vi "Convert Write ERD List to Message.vi"(0 "GEA Inputs":T1 {"Destination" format="%.0x"; "Source" format="%.0x"}, 7 "Write ERD List":T3(array[cluster]) {"ERD Number" format="%.0x"}, 11 "Error In":errorcluster) -> (4 "GEA Message":T2 {"Command" format="%02x"; "Destination" format="%02x"; "Source" format="%02x"}, 15 "Error Out":errorcluster)   [LabVIEW 2023]
doc: "This vi uses the Source / Destination from the GEA input and the ERD Write list to format a single GEA2 message to read the list of ERDs."
uses:
  type defs/Data In.ctl
  type defs/Source_Destination.ctl
  <vilib>/regexp/Match Regular Expression.xnode
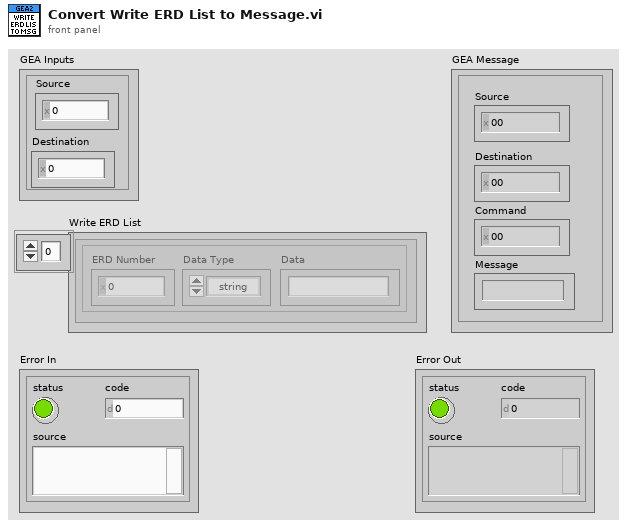
[diagram p1: front panel]
types:
  T1 = typedef "Source_Destination.ctl" = cluster{"Source":u8, "Destination":u8}
  T2 = typedef "Data In.ctl" = cluster{"Source":u8, "Destination":u8, "Command":u8, "Message":string}
  T3 = cluster{"ERD Number":u16, "Data Type":enum16{"string", "boolean", "uint8_t", "uint16_t", "uint32_t", "uint64_t", "int8_t", "int16_t", "int32_t", "int64_t"}, "Data":string}[]
  T4 = enum16{"string", "boolean", "uint8_t", "uint16_t", "uint32_t", "uint64_t", "int8_t", "int16_t", "int32_t", "int64_t"}
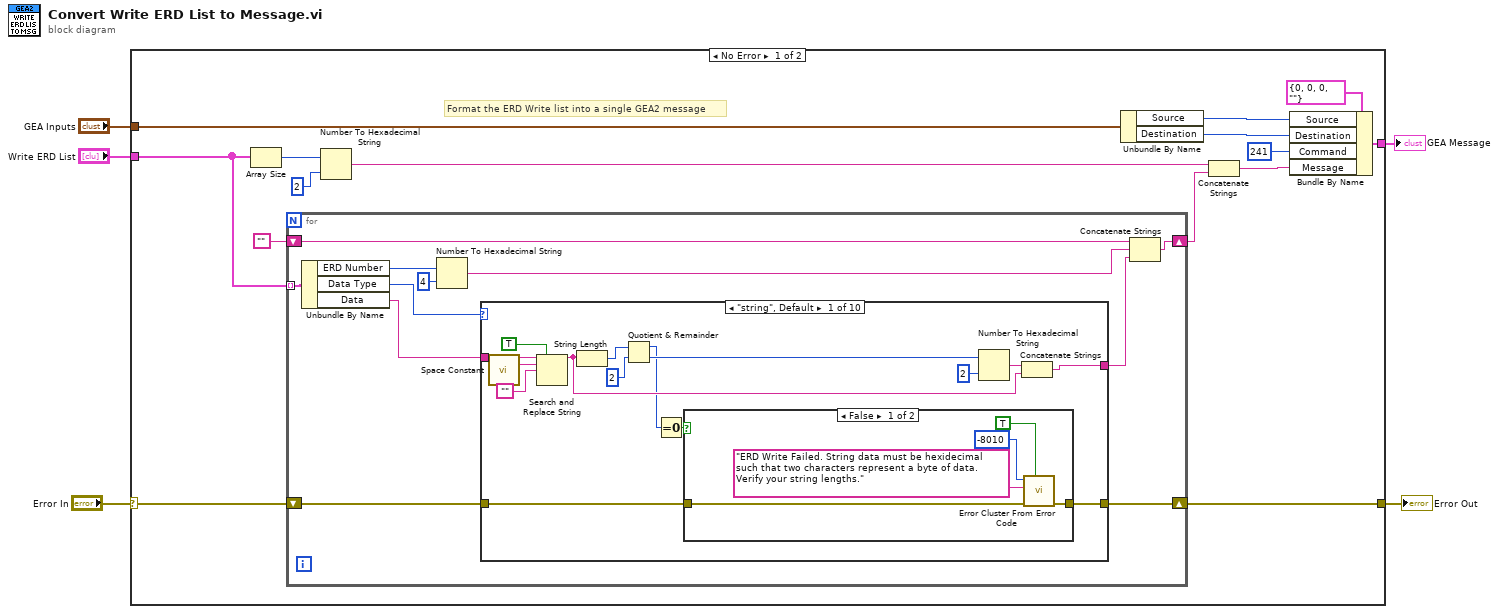
[diagram p0: block diagram]
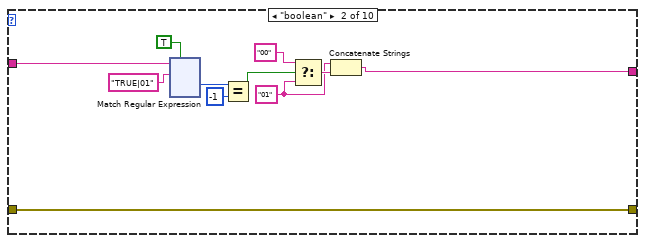
[diagram p3: hidden frame]
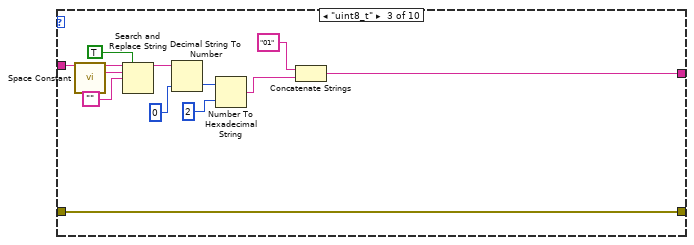
[diagram p4: hidden frame]
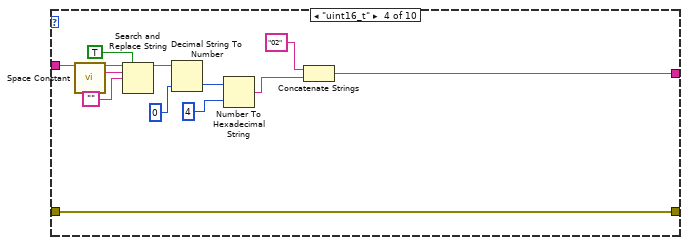
[diagram p5: hidden frame]
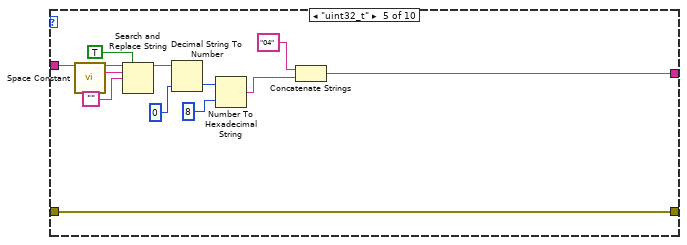
[diagram p6: hidden frame]
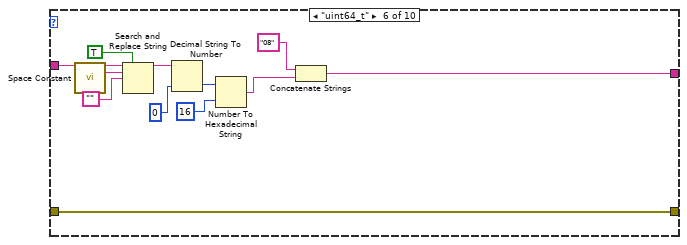
[diagram p7: hidden frame]
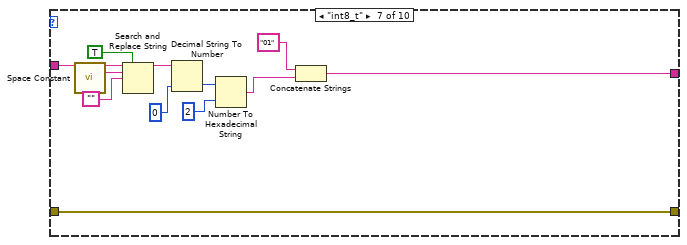
[diagram p8: hidden frame]
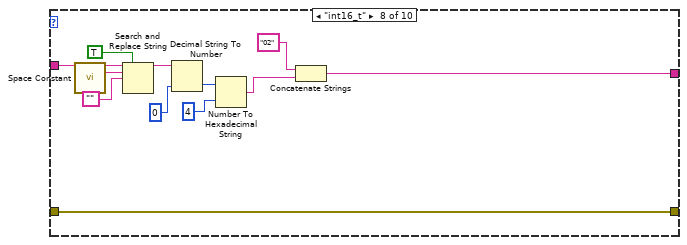
[diagram p9: hidden frame]
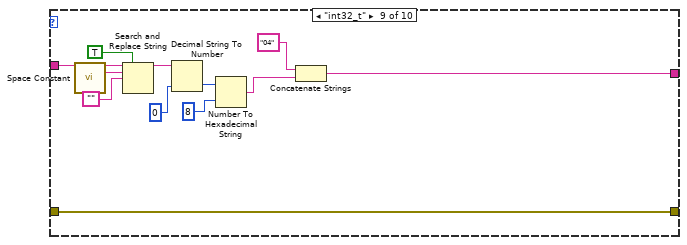
[diagram p10: hidden frame]
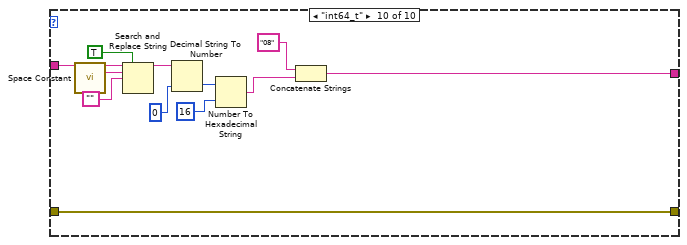
[diagram p11: hidden frame]
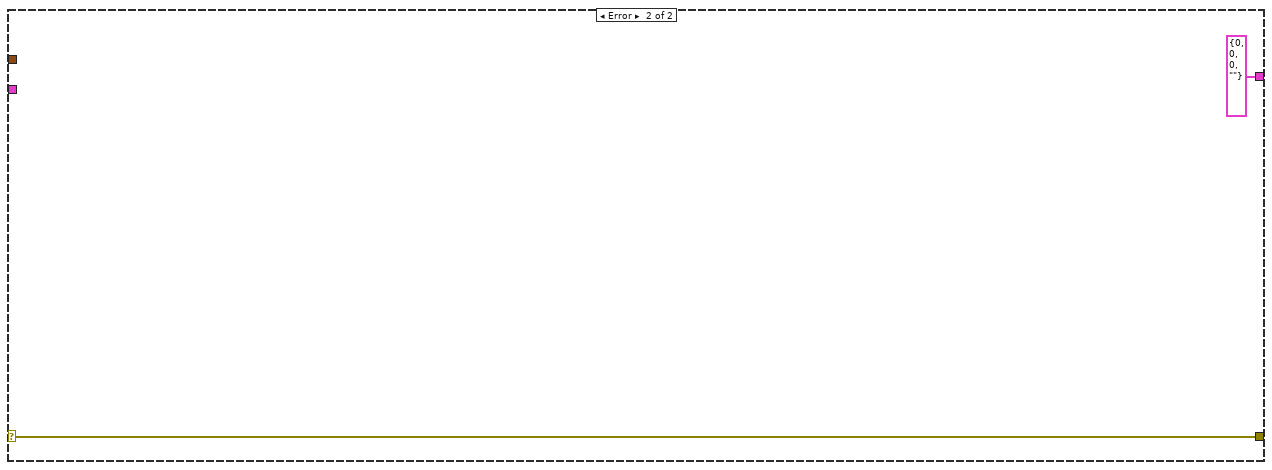
[diagram p12: hidden frame]
diagram:
  n1 = case shown="No Error" "Error In" {
    selector: "Error In" -> [w7 w278]
    tunnel: "Write ERD List" -> [w17 _]
    tunnel: "GEA Inputs" -> [w13 _]
    tunnel: [w8 T2 {"Source"=0, "Destination"=0, "Command"=0, "Message"=""} ("GEA Message")] -> w3
    tunnel: [w6 w278] -> w1
    frame No Error {
      # "Format the ERD Write list into a single GEA2 message"
      n2 = Array Size(array=w17) -> (size(s)=w19:i32)
      n3 = for {
        tunnel: w17 -> [w31] mode=indexing
        shift-right: [w26] -> w15
        shift-left: "" -> [w28]
        shift-right: [w21] -> w6
        shift-left: w7 -> [w22]
        n4 = Unbundle By Name(w31) -> ("ERD Number"=w30:u16, "Data Type"=w25:T4, "Data"=w24:string)
        n5 = Number To Hexadecimal String(1:i16 4 ("width (-)"), 2:w30) -> (0:w27:string)
        n6 = case shown="\"string\", Default" w25 {
          tunnel: w24 -> [w46 w62 w189 w194 w207 w219 w231 w243 w255 w267]
          tunnel: [w41 w55 w188 w195 w206 w218 w230 w242 w254 w266] -> w23
          tunnel: w22 -> [w35 w53 w181 w193 w205 w217 w229 w241 w253 w265]
          tunnel: [w32 w53 w181 w193 w205 w217 w229 w241 w253 w265] -> w21
          frame "string", Default {
            n7 = call <vilib>:"Space Constant.vi"() -> ("String"=w44:string)
            n8 = Search and Replace String(replace all?=TRUE ("replace all? (F)"), input string=w46, search string=w44, replace string="") -> (result string=w40:string)  [unwired: 4 in, 3 out]
            n9 = String Length(string=w40) -> (length=w38:i32)
            n10 = Quotient & Remainder(x=w38, y=2) -> (x-y*floor(x/y)=w34:i32, floor(x/y)=w37:i32)
            n11 = Equal To 0?(x=w34) -> (x = 0?=w33:bool)
            n12 = case shown="False" w33 {
              tunnel: w35 -> [w51 w52]
              tunnel: [w47 w52] -> w32
              frame False {
                n13 = call <vilib>:"Error Cluster From Error Code.vi"("show call chain? (False)"=TRUE, "error in (no error)"=w51, "error message (\"\")"="ERD Write Failed. String data must be hexidecimal such that two characters represent a byte of data. Verify your string lengths." ("error message (\"\")"), "error code (0)"=-8010) -> ("error out"=w47:errorcluster)  [unwired: 5 in]
              }
              frame True {
              }
            }
            n14 = Number To Hexadecimal String(1:i16 2 ("width (-)"), 2:w37) -> (0:w42:string)
            n15 = Concatenate Strings(w42, w40) -> (w41:string)
          }
          frame "boolean" {
            w54 = "01"
            n16 = xnode "Match Regular Expression"("input string"=w62, "regular expression"="TRUE|01", "ignore case? (F)"=TRUE) -> ("offset past match"=w60:i32)  [unwired: 3 in, 4 out]
            n17 = Equal?(x=w60, y=-1) -> (x = y?=w57:bool)
            n18 = Select(t="00", s=w57, f=w54) -> (s? t:f=w56:string)
            n19 = Concatenate Strings(w54, w56) -> (w55:string)
          }
          frame "uint8_t" {
            n20 = call <vilib>:"Space Constant.vi"() -> ("String"=w191:string)
            n21 = Search and Replace String(replace all?=TRUE ("replace all? (F)"), input string=w189, search string=w191, replace string="") -> (result string=w186:string)  [unwired: 4 in, 3 out]
            n22 = Decimal String To Number(string=w186, default (0L)=u8 0) -> (number=w183:u8)  [unwired: 1 in, 1 out]
            n23 = Number To Hexadecimal String(1:i16 2 ("width (-)"), 2:w183) -> (0:w182:string)
            n24 = Concatenate Strings("01", w182) -> (w188:string)
          }
          frame "uint16_t" {
            n25 = call <vilib>:"Space Constant.vi"() -> ("String"=w203:string)
            n26 = Search and Replace String(replace all?=TRUE ("replace all? (F)"), input string=w194, search string=w203, replace string="") -> (result string=w200:string)  [unwired: 4 in, 3 out]
            n27 = Decimal String To Number(string=w200, default (0L)=u16 0) -> (number=w197:u16)  [unwired: 1 in, 1 out]
            n28 = Number To Hexadecimal String(1:i16 4 ("width (-)"), 2:w197) -> (0:w196:string)
            n29 = Concatenate Strings("02", w196) -> (w195:string)
          }
          frame "uint32_t" {
            n30 = call <vilib>:"Space Constant.vi"() -> ("String"=w215:string)
            n31 = Search and Replace String(replace all?=TRUE ("replace all? (F)"), input string=w207, search string=w215, replace string="") -> (result string=w212:string)  [unwired: 4 in, 3 out]
            n32 = Decimal String To Number(string=w212, default (0L)=u32 0) -> (number=w209:u32)  [unwired: 1 in, 1 out]
            n33 = Number To Hexadecimal String(1:i16 8 ("width (-)"), 2:w209) -> (0:w208:string)
            n34 = Concatenate Strings("04", w208) -> (w206:string)
          }
          frame "uint64_t" {
            n35 = call <vilib>:"Space Constant.vi"() -> ("String"=w227:string)
            n36 = Search and Replace String(replace all?=TRUE ("replace all? (F)"), input string=w219, search string=w227, replace string="") -> (result string=w224:string)  [unwired: 4 in, 3 out]
            n37 = Decimal String To Number(string=w224, default (0L)=u64 0) -> (number=w221:u64)  [unwired: 1 in, 1 out]
            n38 = Number To Hexadecimal String(1:i16 16 ("width (-)"), 2:w221) -> (0:w220:string)
            n39 = Concatenate Strings("08", w220) -> (w218:string)
          }
          frame "int8_t" {
            n40 = call <vilib>:"Space Constant.vi"() -> ("String"=w239:string)
            n41 = Search and Replace String(replace all?=TRUE ("replace all? (F)"), input string=w231, search string=w239, replace string="") -> (result string=w236:string)  [unwired: 4 in, 3 out]
            n42 = Decimal String To Number(string=w236, default (0L)=i8 0) -> (number=w233:i8)  [unwired: 1 in, 1 out]
            n43 = Number To Hexadecimal String(1:i16 2 ("width (-)"), 2:w233) -> (0:w232:string)
            n44 = Concatenate Strings("01", w232) -> (w230:string)
          }
          frame "int16_t" {
            n45 = call <vilib>:"Space Constant.vi"() -> ("String"=w251:string)
            n46 = Search and Replace String(replace all?=TRUE ("replace all? (F)"), input string=w243, search string=w251, replace string="") -> (result string=w248:string)  [unwired: 4 in, 3 out]
            n47 = Decimal String To Number(string=w248, default (0L)=i16 0) -> (number=w245:i16)  [unwired: 1 in, 1 out]
            n48 = Number To Hexadecimal String(1:i16 4 ("width (-)"), 2:w245) -> (0:w244:string)
            n49 = Concatenate Strings("02", w244) -> (w242:string)
          }
          frame "int32_t" {
            n50 = call <vilib>:"Space Constant.vi"() -> ("String"=w263:string)
            n51 = Search and Replace String(replace all?=TRUE ("replace all? (F)"), input string=w255, search string=w263, replace string="") -> (result string=w260:string)  [unwired: 4 in, 3 out]
            n52 = Decimal String To Number(string=w260, default (0L)=0) -> (number=w257:i32)  [unwired: 1 in, 1 out]
            n53 = Number To Hexadecimal String(1:i16 8 ("width (-)"), 2:w257) -> (0:w256:string)
            n54 = Concatenate Strings("04", w256) -> (w254:string)
          }
          frame "int64_t" {
            n55 = call <vilib>:"Space Constant.vi"() -> ("String"=w275:string)
            n56 = Search and Replace String(replace all?=TRUE ("replace all? (F)"), input string=w267, search string=w275, replace string="") -> (result string=w272:string)  [unwired: 4 in, 3 out]
            n57 = Decimal String To Number(string=w272, default (0L)=i64 0) -> (number=w269:i64)  [unwired: 1 in, 1 out]
            n58 = Number To Hexadecimal String(1:i16 16 ("width (-)"), 2:w269) -> (0:w268:string)
            n59 = Concatenate Strings("08", w268) -> (w266:string)
          }
        }
        n60 = Concatenate Strings(w28, w27, w23) -> (w26:string)
      }
      n61 = Number To Hexadecimal String(1:i16 2 ("width (-)"), 2:w19) -> (0:w18:string)
      n62 = Unbundle By Name(w13) -> ("Source"=w12:u8, "Destination"=w11:u8)
      n63 = Concatenate Strings(w18, w15) -> (w9:string)
      n64 = Bundle By Name(cluster=T2 {"Source"=0, "Destination"=0, "Command"=0, "Message"=""} ("GEA Message"), "Source"=w12, "Destination"=w11, "Command"=u8 241, "Message"=w9) -> (w8:T2)
    }
    frame Error {
    }
  }
  "GEA Message" <- w3
  "Error Out" <- w1
